vi "Reconfig ECAT Modules.vi"(8 "error in (no error)":errorcluster) -> (0 "error out":errorcluster)   [LabVIEW 2016, in "Scan Engine Custom Device.lvlib"]
uses:
  Scan Engine Custom Device.lvlib
  Type Defs/ECAT Reconfig State.ctl
  Modules.lvlibp/RSI Module/RSI Module.lvclass
  Type Defs/ECAT Module Reconfig.ctl
  Type Defs/ECAT Reconfig Status.ctl
panel:
  in  "Status":refnum<queue>
  in  "ECAT Modules":T1[](array[typedef])
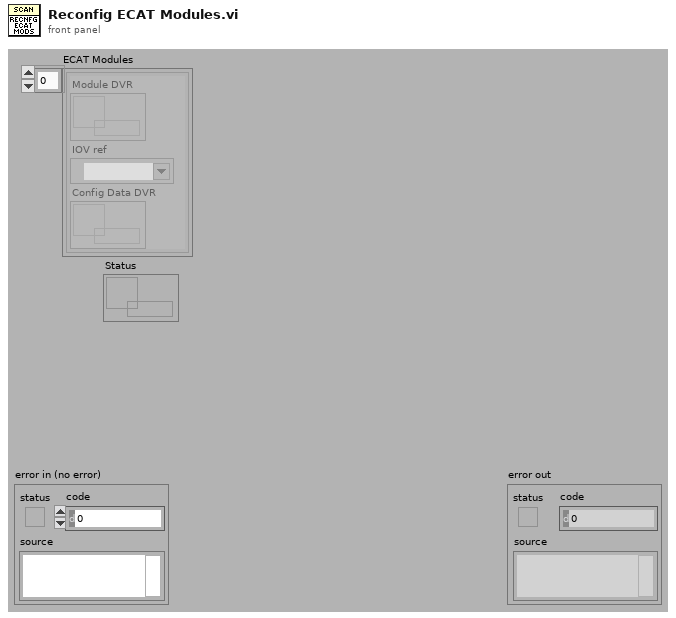
[diagram p1: front panel]
types:
  T1 = typedef "Scan Engine Custom Device.lvlib/ECAT Module Reconfig.ctl" = cluster{"Module DVR":refnum<data-value>, "IOV ref":refnum<k21>, "Config Data DVR":refnum<data-value>}
  T2 = typedef "Scan Engine Custom Device.lvlib/ECAT Reconfig State.ctl" = enum16{"Not running", "Waiting to Start", "Started", "Running"}
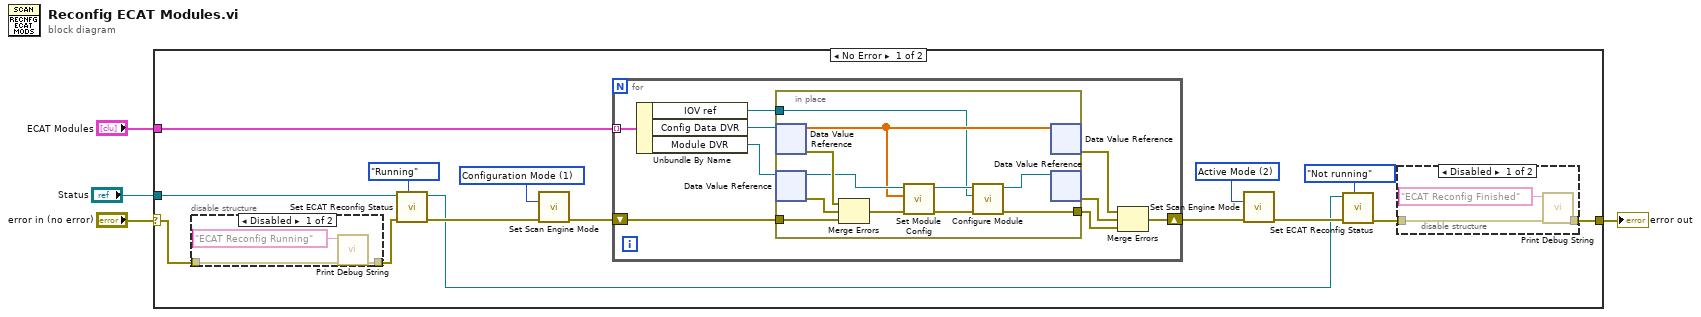
[diagram p0: block diagram]
diagram:
  n1 = case shown="No Error" "error in (no error)" {
    selector: "error in (no error)" -> [w6 w48]
    tunnel: "ECAT Modules" -> [w19 _]
    tunnel: [w7 w48] -> w2
    tunnel: "Status" -> [w13 _]
    frame No Error {
      w15 = 2 items=["Configuration Mode"=1, "Active Mode"=2] ("mode (Active Mode)")
      w18 = 1 items=["Configuration Mode"=1, "Active Mode"=2] ("mode (Active Mode)")
      n2 = disable-structure shown="Disabled" {
        disable-tunnel: w6 -> [w25 w27]
        disable-tunnel: [w24 w27] -> w5
        frame Disabled {
          n3 = call "Print Debug String.vi"("error in"=w25, "String to write"="ECAT Reconfig Running") -> ("error out"=w24:errorcluster)  [unwired: 8 in]
        }
        frame Enabled {
        }
      }
      n4 = call "Set ECAT Reconfig Status.vi"("State"=ECAT_Reconfig_State."Running", "error in (no error)"=w5, "Status in"=w13) -> ("error out"=w14:errorcluster, "Status out"=w9:refnum<queue>)  [unwired: 7 in]
      n5 = call <vilib>:"Set Scan Engine Mode.vi"("mode (Active Mode)"=w18, "error in (no error)"=w14) -> ("error out"=w17:errorcluster)  [unwired: 13 in]
      n6 = for {
        tunnel: w19 -> [w36] mode=indexing
        shift-right: [w31] -> w16
        shift-left: w17 -> [w33]
        n7 = Unbundle By Name(w36) -> ("IOV ref"=w32:refnum<k21>, "Config Data DVR"=w35:refnum<data-value>, "Module DVR"=w34:refnum<data-value>)
        n8 = in-place {
          in-place-border: w33 -> [w47]
          in-place-border: w32 -> [w37]
          in-place-border: [w38] -> w28
          n9 = in-place-dvr #1(w35) -> (w39:dbl[], w45:errorcluster)
          n10 = in-place-dvr #2(w34) -> (w41:refnum<class "RSI Module.lvclass">, w46:errorcluster)
          n11 = Merge Errors(w45, w46, w47) -> (w42:errorcluster)
          n12 = call-dynamic "Set Module Config.vi"("error in (no error)"=w42, "Config Channels"=w39, "RSI Module in"=w41) -> ("error out"=w43:errorcluster, "RSI Module out"=w44:refnum<class "RSI Module.lvclass">)  [unwired: 7 in]
          n13 = call-dynamic "Configure Module.vi"("error in (no error)"=w43, "IOV ref in"=w37, "RSI Module in"=w44) -> ("error out"=w38:errorcluster, "RSI Module out"=w40:refnum<class "RSI Module.lvclass">)  [unwired: 6 in, 1 out]
          n14 = in-place-dvr #1(w39) -> (w30:errorcluster)  [unwired: 1 out]
          n15 = in-place-dvr #2(w40) -> (w29:errorcluster)  [unwired: 1 out]
        }
        n16 = Merge Errors(w30, w29, w28) -> (w31:errorcluster)
      }
      n17 = call <vilib>:"Set Scan Engine Mode.vi"("mode (Active Mode)"=w15, "error in (no error)"=w16) -> ("error out"=w10:errorcluster)  [unwired: 13 in]
      n18 = call "Set ECAT Reconfig Status.vi"("State"=ECAT_Reconfig_State."Not running", "error in (no error)"=w10, "Status in"=w9) -> ("error out"=w8:errorcluster)  [unwired: 7 in, 1 out]
      n19 = disable-structure shown="Disabled" {
        disable-tunnel: w8 -> [w21 w23]
        disable-tunnel: [w20 w23] -> w7
        frame Disabled {
          n20 = call "Print Debug String.vi"("error in"=w21, "String to write"="ECAT Reconfig Finished") -> ("error out"=w20:errorcluster)  [unwired: 8 in]
        }
        frame Enabled {
        }
      }
    }
    frame Error {
    }
  }
  "error out" <- w2
